vi "initialise.vi"(8 "error in (no error)":errorcluster, 11 "BalloonNotifier in":refnum<class "BalloonNotifier.lvclass">) -> (0 "error out":errorcluster, 3 "BalloonNotifier out":refnum<class "BalloonNotifier.lvclass">)   [LabVIEW 2010, in "BalloonNotifier.lvclass"]
uses:
  BalloonNotifier.lvclass
  balloon_events.ctl
  balloon_event_registration_actions.ctl
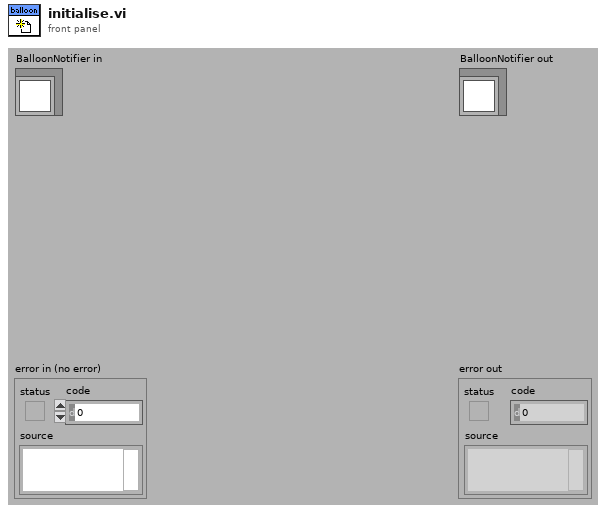
[diagram p1: front panel]
types:
  T1 = typedef "BalloonNotifier.lvclass/balloon_event_registration_actions.ctl" = enum16{"Initial Event Registration", "Add to Event Registration", "Destroy Events and Re-register"}
  T2 = typedef "BalloonNotifier.lvclass/balloon_events.ctl" = enum16{"BalloonTipClicked", "BalloonTipClosed", "BalloonTipShown", "Click", "Disposed", "DoubleClick", "MouseClick", "MouseDoubleClick", "MouseDown", "MouseMove", "MouseUp", "MenuItemClick", "MenuItemSelect"}
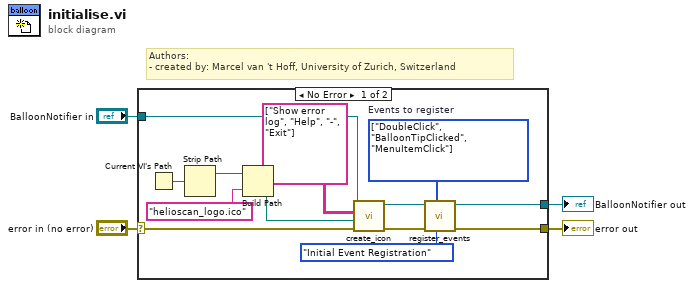
[diagram p0: block diagram]
diagram:
  # "Authors: \n- created by: Marcel van 't Hoff, University of Zurich, Switzerland"
  n1 = case shown="No Error" "error in (no error)" {
    selector: "error in (no error)" -> [w14 w19]
    tunnel: [w5 w19] -> w3
    tunnel: [w6 w18] -> w1
    tunnel: "BalloonNotifier in" -> [w11 w18]
    frame No Error {
      w7 = T2[] [enum."DoubleClick", enum."BalloonTipClicked", enum."MenuItemClick"] items=["BalloonTipClicked", "BalloonTipClosed", "BalloonTipShown", "Click", "Disposed", "DoubleClick", "MouseClick", "MouseDoubleClick", "MouseDown", "MouseMove", "MouseUp", "MenuItemClick", "MenuItemSelect"]  # Events to register
      n2 = Current VI's Path() -> (path=w17:path)
      n3 = Strip Path(path=w17) -> (stripped path=w16:path)  [unwired: 1 out]
      n4 = Build Path(base path=w16, name or relative path="helioscan_logo.ico") -> (appended path=w12:path)
      n5 = call-dynamic "create_icon.vi"("error in (no error)"=w14, "Icon File Path"=w12, "Context Menu (optional)"=string[][] [["Show error log"], ["Help"], ["-"], ["Exit"]], "BalloonNotifier in"=w11) -> ("error out"=w9:errorcluster, "BalloonNotifier out"=w8:refnum<class "BalloonNotifier.lvclass">)  [unwired: 6 in]
      n6 = call-dynamic "register_events.vi"("Action"=balloon_event_registration_actions."Initial Event Registration", "Events to register"=w7, "error in (no error)"=w9, "BalloonNotifier in"=w8) -> ("error out"=w5:errorcluster, "BalloonNotifier out"=w6:refnum<class "BalloonNotifier.lvclass">)  [unwired: 6 in]
    }
    frame Error {
    }
  }
  "error out" <- w3
  "BalloonNotifier out" <- w1
